vi "tcp tx.vi"(8 "error in":errorcluster, 9 "timeout ms (5000)":i32=5000, 10 "tx":string, 11 "TCP Connection in":refnum<k5>) -> (0 "error out":errorcluster, 3 "TCP Connection out":refnum<k5>)   [LabVIEW 2014]
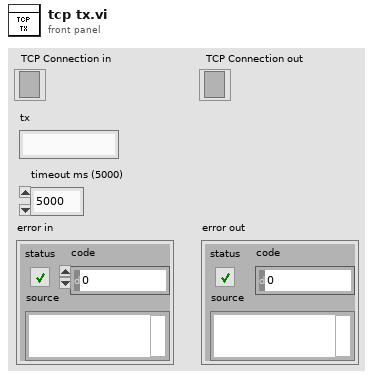
[diagram p1: front panel]
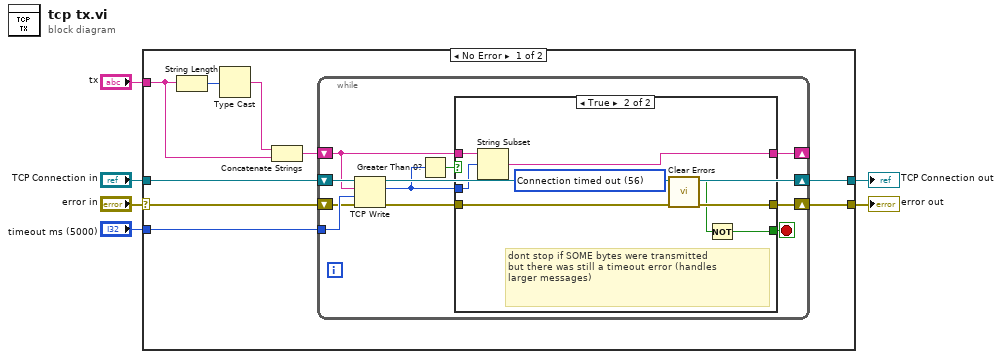
[diagram p0: block diagram]
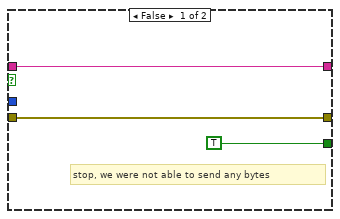
[diagram p2: hidden frame]
diagram:
  n1 = case shown="No Error" "error in" {
    selector: "error in" -> [w7 w39]
    tunnel: "timeout ms (5000)" -> [w15 _]
    tunnel: [w14 w38] -> w5
    tunnel: "TCP Connection in" -> [w13 w38]
    tunnel: "tx" -> [w9 _]
    tunnel: [w8 w39] -> w2
    frame No Error {
      n2 = String Length(string=w9) -> (length=w10:i32)
      n3 = Type Cast(x=w10) -> (*(type *) &x=w11:string)  [unwired: 1 in]
      n4 = Concatenate Strings(w11, w9) -> (w12:string)
      n5 = while {
        tunnel: w15 -> [w26]
        shift-right: [w25] -> w14
        shift-left: w13 -> [w24]
        shift-right: [w19] -> w8
        shift-left: w7 -> [w23]
        shift-right: [w21] -> _
        shift-left: w12 -> [w22]
        stop <- w16 stop-if-true
        n6 = TCP Write(connection ID=w24, data in=w22, error in (no error)=w23, 9:w26) -> (connection ID out=w25:refnum<k5>, bytes written=w18:i32, error out=w20:errorcluster)
        n7 = Greater Than 0?(x=w18) -> (x > 0?=w17:bool)
        n8 = case shown="True" w17 {
          tunnel: w22 -> [w28 w37]
          tunnel: w18 -> [_ w36]
          tunnel: [w28 w35] -> w21
          tunnel: w20 -> [w29 w33]
          tunnel: [w29 w32] -> w19
          tunnel: [TRUE w31] -> w16
          frame False {
            # "stop, we were not able to send any bytes"
          }
          frame True {
            w34 = 56 items=["No Error", "Argument Error", "Memory Full", "Out of Zone", "End of File", "File Already Open", "Generic File IO Error", "File Not Found", "File Permission Error", "Disk Full", "Duplicate Path", "Too Many Files Open", "Not Enabled", "Resource File Not Found", "Cannot Add Resource", "Resource Not Found", "Image Not Found", "Image Memory Error", "Pen Does Not Exist", "Config Bad Type", "Config Token Not Found", "Config Parse Error", "Config Memory Error", "Bad External Code Format", "Bad External Code Offset", "External Code Not Present", "Null Window", "Destroy Window Mixup", "Null Menu", "Print Aborted", "Bad Print Record", "Print Driver Error", "Windows Error During Print", "Memory Error During Print", "Print Dialog Error", "Generic Print Error", "Invalid Device Refnum", "Device Not Found", "Device Parameter Error", "Device Unit Error", "Can't Open Device", "Device Call Aborted", "Generic Error", "Cancelled By User", "Object ID Too Low", "Object ID Too High", "Object Not In Heap", "Unknown Heap", "Bad DefProc ID", "DefProc Not In Table", "Message Out Of Range", "Null Method", "Unknown Message", "Manager Call Not Supported", "Bad address", "Connection In progress", "Connection timed out", "Connection is already in progress", "Network attribute not supported", "Network error", "Address in use", "System out of memory", "Connection aborted", "Connection refused", "Connection is not connected", "Connection is already connected", "Connection closed", "Initialize error (interapplication manager)", "Bad occurrence", "Wait on unbound occurrence handler", "Occurrence queue overflow", "Bad path", "Semaphore not signaled", "Unrecognized type (interapplication manager)"] ("1st Error to Convert")
            # "dont stop if SOME bytes were transmitted\nbut there was still a timeout error (handles\nlarger messages)"
            n9 = String Subset(string=w37, offset (0)=w36) -> (substring=w35:string)  [unwired: 1 in]
            n10 = call <vilib>:"Clear Errors.vi"("error in (no error)"=w33, "specific error code to clear (0: all)"=w34) -> ("error out"=w32:errorcluster, "specific error cleared?"=w30:bool)  [unwired: 4 in]
            n11 = Not(x=w30) -> (.not. x?=w31:bool)
          }
        }
      }
    }
    frame Error {
    }
  }
  "TCP Connection out" <- w5
  "error out" <- w2
